vi "ramseywaveformprepareRFcoil.vi"(6 "RF pulse length (Units 1us)":dbl=1000.0, 9 "1762 pulse length (units of 1 us)":dbl=50.0) -> (3 "digital waveform out 2":digitalwaveform(waveform)={"t0"=timestamp(0 s since 1904-01-01), "dt"=1e-07, "Y"={"transitions"=[0, 2100, 2200, 2300, 2351, 2401, 2451, 2551], "data"=[[0, 1, 1, 1, 0, 0], [0, 1, 0, 1, 0, 0], [0, 1, 0, 0, 0, 0], [0, 0, 0, 0, 0, 0], [1, 0, 0, 0, 0, 0], [0, 0, 0, 0, 0, 1], [0, 0, 0, 0, 0, 0], [0, 0, 1, 1, 0, 0]]}, "error"={"status"=FALSE, "code"=37421928, "source"=""}})   [LabVIEW 2012]
uses:
  <vilib>/Waveform/DWDTOps.llb/Digital Pattern Generator (Single Value).vi
  <vilib>/Waveform/DWDTOps.llb/DWDT Append Digital Samples.vi
panel:
  out "Mixed Signal Graph":digitalwaveform(graph)={"t0"=timestamp(0 s since 1904-01-01), "dt"=1e-07, "Y"={"transitions"=[0, 2100, 2200, 2300, 2351, 2401, 2451, 2551], "data"=[[0, 1, 1, 1, 0, 0], [0, 1, 0, 1, 0, 0], [0, 1, 0, 0, 0, 0], [0, 0, 0, 0, 0, 0], [1, 0, 0, 0, 0, 0], [0, 0, 0, 0, 0, 1], [0, 0, 0, 0, 0, 0], [0, 0, 1, 1, 0, 0]]}, "error"={"status"=FALSE, "code"=37421928, "source"=""}}
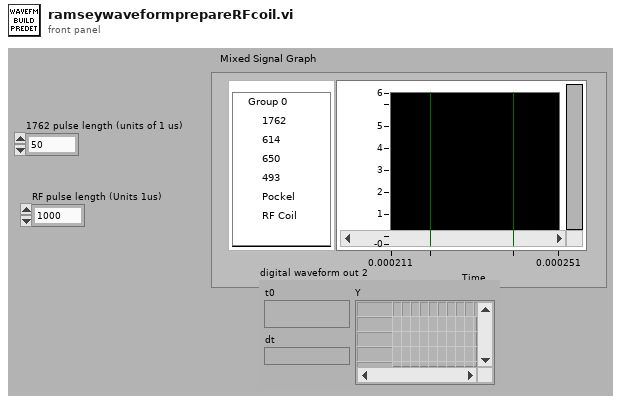
[diagram p1: front panel]
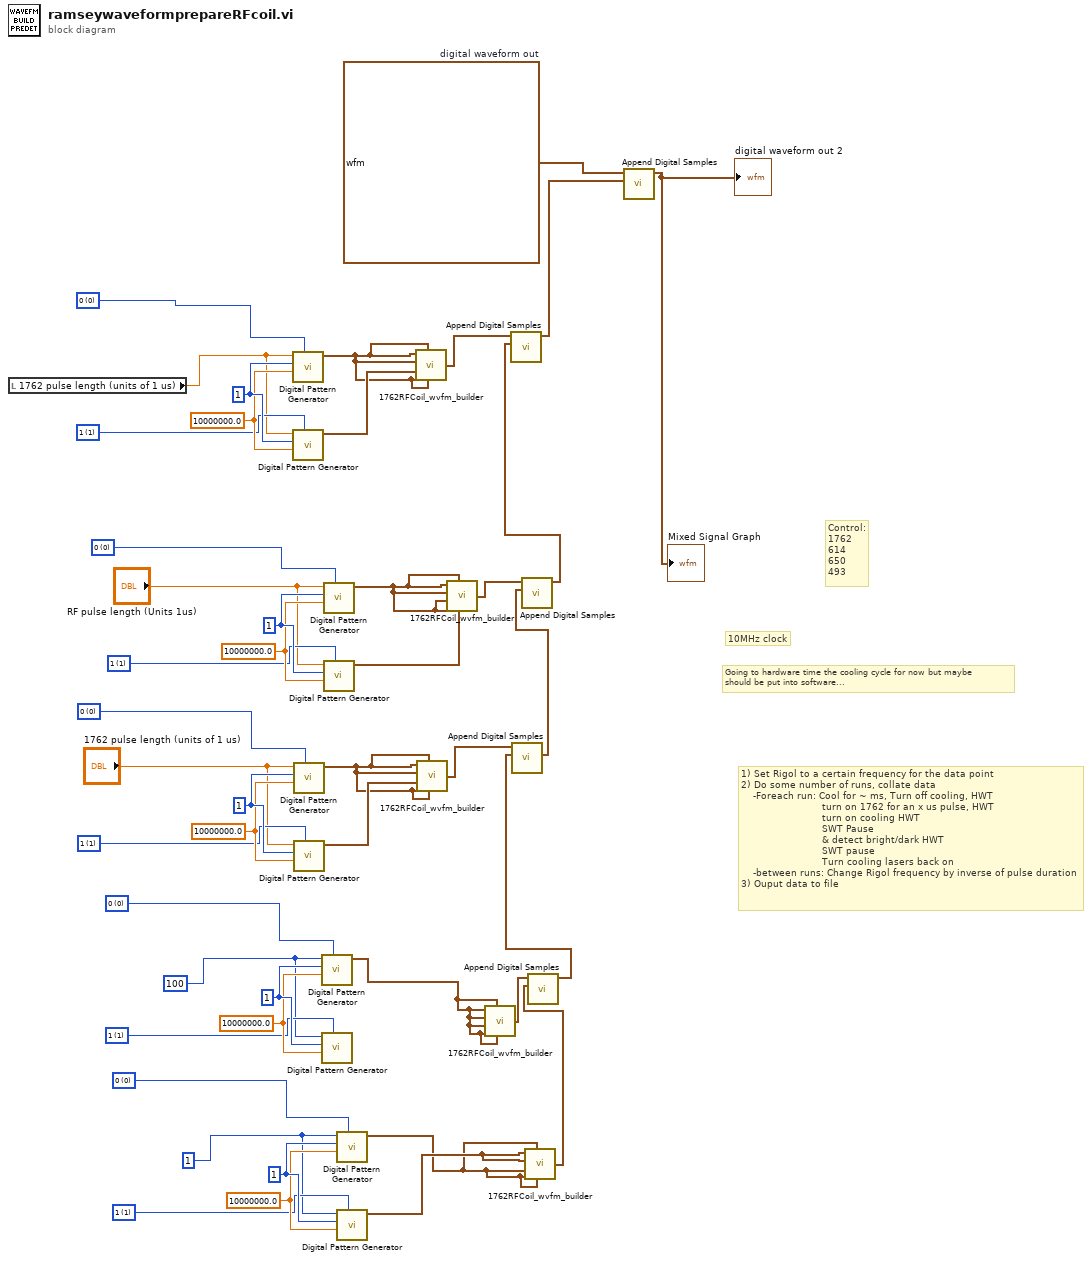
[diagram p0: block diagram]
diagram:
  w2 = u8 0 items=["0", "1", "Z", "L", "H", "X", "T", "V"] ("value")
  w10 = u32 1 ("number of signals")
  w8 = u8 1 items=["0", "1", "Z", "L", "H", "X", "T", "V"] ("value")
  w9 = 10000000.0 ("rate")
  w19 = u8 0 items=["0", "1", "Z", "L", "H", "X", "T", "V"] ("value")
  w18 = u32 1 ("number of signals")
  w16 = u8 1 items=["0", "1", "Z", "L", "H", "X", "T", "V"] ("value")
  w17 = 10000000.0 ("rate")
  w29 = u32 1 ("number of samples")
  w33 = u8 0 items=["0", "1", "Z", "L", "H", "X", "T", "V"] ("value")
  w32 = u32 1 ("number of signals")
  w30 = u8 1 items=["0", "1", "Z", "L", "H", "X", "T", "V"] ("value")
  w31 = 10000000.0 ("rate")
  w34 = u32 100 ("number of samples")
  w38 = u8 0 items=["0", "1", "Z", "L", "H", "X", "T", "V"] ("value")
  w37 = u32 1 ("number of signals")
  w35 = u8 1 items=["0", "1", "Z", "L", "H", "X", "T", "V"] ("value")
  w36 = 10000000.0 ("rate")
  w45 = u8 0 items=["0", "1", "Z", "L", "H", "X", "T", "V"] ("value")
  w44 = u32 1 ("number of signals")
  w42 = u8 1 items=["0", "1", "Z", "L", "H", "X", "T", "V"] ("value")
  w43 = 10000000.0 ("rate")
  w39 = digitalwaveform {"t0"=timestamp(0 s since 1904-01-01), "dt"=1e-07, "Y"={"transitions"=[0, 2100, 2200, 2300, 2350], "data"=[[0, 1, 1, 1, 0, 0], [0, 1, 0, 1, 0, 0], [0, 1, 0, 0, 0, 0], [0, 0, 0, 0, 0, 0], [0, 0, 0, 0, 0, 0]]}, "error"={"status"=FALSE, "code"=37421928, "source"=""}}  # digital waveform out
  # "Going to hardware time the cooling cycle for now but maybe\nshould be put into software..."
  # "10MHz clock"
  # "Control:\n1762\n614\n650\n493"
  # "1) Set Rigol to a certain frequency for the data point\n2) Do some number of runs, collate data\n    -Foreach run: Cool for ~ ms, Turn off cooling, HWT\n                           turn on 1762 for an x us pulse, HWT\n                           turn on cooling HWT\n                           SWT Pause\n                           & detect bright/dark HWT\n                           SWT pause\n                           Turn cooling lasers back on \n    -between runs: Change Rigol frequency by inverse of pulse duration\n3) Ouput data to file"
  n1 = local read "1762 pulse length (units of 1 us)"() -> (w1:dbl)
  n2 = call-poly <vilib>:"Digital Pattern Generator.vi"("value"=w2, "sample rate"=w9, "number of signals"=w10, "number of samples"=w1) -> ("digital waveform"=w5:digitalwaveform)  [unwired: 6 in, 1 out]
  n3 = call-poly <vilib>:"Digital Pattern Generator.vi"("value"=w8, "sample rate"=w9, "number of signals"=w10, "number of samples"=w1) -> ("digital waveform"=w6:digitalwaveform)  [unwired: 6 in, 1 out]
  n4 = call-poly <vilib>:"Digital Pattern Generator.vi"("value"=w45, "sample rate"=w43, "number of signals"=w44, "number of samples"="1762 pulse length (units of 1 us)") -> ("digital waveform"=w22:digitalwaveform)  [unwired: 6 in, 1 out]
  n5 = call-poly <vilib>:"Digital Pattern Generator.vi"("value"=w42, "sample rate"=w43, "number of signals"=w44, "number of samples"="1762 pulse length (units of 1 us)") -> ("digital waveform"=w23:digitalwaveform)  [unwired: 6 in, 1 out]
  n6 = call-poly <vilib>:"Digital Pattern Generator.vi"("value"=w38, "sample rate"=w36, "number of signals"=w37, "number of samples"=w34) -> ("digital waveform"=w21:digitalwaveform)  [unwired: 6 in, 1 out]
  n7 = call-poly <vilib>:"Digital Pattern Generator.vi"("value"=w35, "sample rate"=w36, "number of signals"=w37, "number of samples"=w34) -> ()  [unwired: 6 in, 2 out]
  n8 = call-poly <vilib>:"Digital Pattern Generator.vi"("value"=w19, "sample rate"=w17, "number of signals"=w18, "number of samples"="RF pulse length (Units 1us)") -> ("digital waveform"=w12:digitalwaveform)  [unwired: 6 in, 1 out]
  n9 = call-poly <vilib>:"Digital Pattern Generator.vi"("value"=w16, "sample rate"=w17, "number of signals"=w18, "number of samples"="RF pulse length (Units 1us)") -> ("digital waveform"=w11:digitalwaveform)  [unwired: 6 in, 1 out]
  n10 = call-poly <vilib>:"Digital Pattern Generator.vi"("value"=w33, "sample rate"=w31, "number of signals"=w32, "number of samples"=w29) -> ("digital waveform"=w20:digitalwaveform)  [unwired: 6 in, 1 out]
  n11 = call-poly <vilib>:"Digital Pattern Generator.vi"("value"=w30, "sample rate"=w31, "number of signals"=w32, "number of samples"=w29) -> ("digital waveform"=w25:digitalwaveform)  [unwired: 6 in, 1 out]
  n12 = call "1762RFCoil_wvfm_builder.vi"("RFCoil"=w5, "pockel"=w5, "614"=w5, "1762"=w6, "650"=w5, "493"=w5) -> ("out"=w7:digitalwaveform)
  n13 = call "1762RFCoil_wvfm_builder.vi"("RFCoil"=w22, "pockel"=w22, "614"=w22, "1762"=w23, "650"=w22, "493"=w22) -> ("out"=w27:digitalwaveform)
  n14 = call "1762RFCoil_wvfm_builder.vi"("RFCoil"=w11, "pockel"=w12, "614"=w12, "1762"=w12, "650"=w12, "493"=w12) -> ("out"=w14:digitalwaveform)
  n15 = call "1762RFCoil_wvfm_builder.vi"("RFCoil"=w21, "pockel"=w21, "614"=w21, "1762"=w21, "650"=w21, "493"=w21) -> ("out"=w26:digitalwaveform)
  n16 = call "1762RFCoil_wvfm_builder.vi"("RFCoil"=w20, "pockel"=w20, "614"=w20, "1762"=w20, "650"=w25, "493"=w25) -> ("out"=w24:digitalwaveform)
  n17 = call-poly <vilib>:"Append Digital Samples.vi"("digital waveform B"=w24, "digital waveform A"=w26) -> ("digital waveform out"=w28:digitalwaveform)  [unwired: 8 in, 1 out]
  n18 = call-poly <vilib>:"Append Digital Samples.vi"("digital waveform B"=w28, "digital waveform A"=w27) -> ("digital waveform out"=w13:digitalwaveform)  [unwired: 8 in, 1 out]
  n19 = call-poly <vilib>:"Append Digital Samples.vi"("digital waveform B"=w13, "digital waveform A"=w14) -> ("digital waveform out"=w3:digitalwaveform)  [unwired: 8 in, 1 out]
  n20 = call-poly <vilib>:"Append Digital Samples.vi"("digital waveform B"=w3, "digital waveform A"=w7) -> ("digital waveform out"=w4:digitalwaveform)  [unwired: 8 in, 1 out]
  n21 = call-poly <vilib>:"Append Digital Samples.vi"("digital waveform B"=w4, "digital waveform A"=w39) -> ("digital waveform out"=→"Mixed Signal Graph" →"digital waveform out 2":digitalwaveform)  [unwired: 8 in, 1 out]
